vi "getAdditionalDataXML.vi"(8 "error in (no error)":errorcluster, 11 "PlayFile in":refnum<class "PlayFile.lvclass">) -> (0 "error out":errorcluster, 2 "additionalDataXML":refnum<class "xmlNode.lvclass">, 3 "PlayFile out":refnum<class "PlayFile.lvclass">)   [LabVIEW 2011, in "Tools.lvlib" / "Scripting.lvlib" / "PlayFile.lvclass"]
uses:
  PlayFile.lvclass
  xmlNode/xmlNode.lvclass
  PlayFile.lvclass/PlayFile.ctl
  ScriptEvent.lvclass
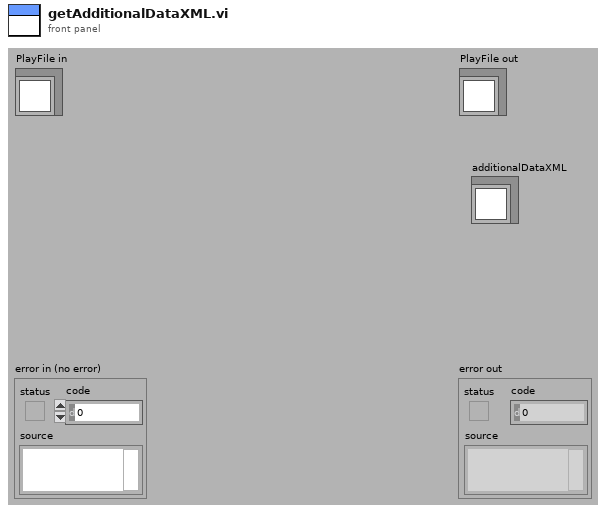
[diagram p1: front panel]
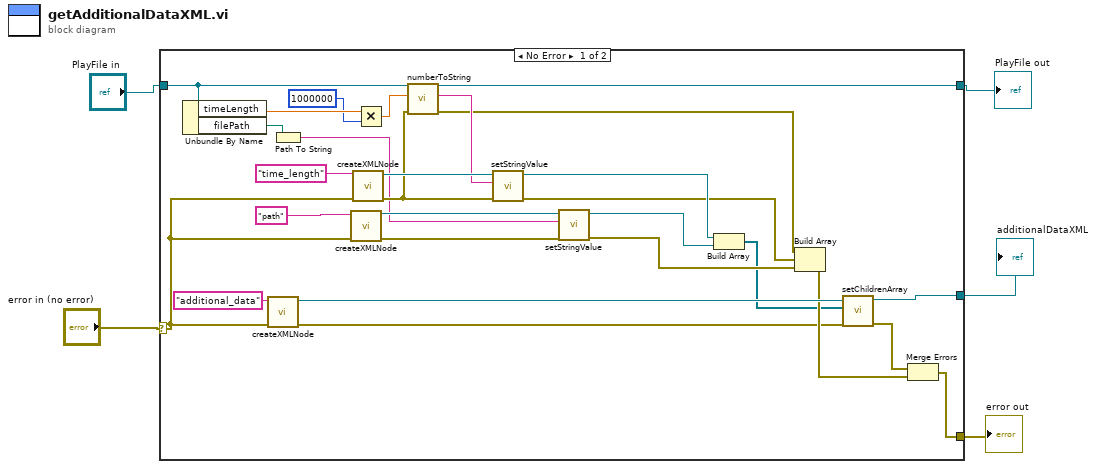
[diagram p0: block diagram]
diagram:
  n1 = case shown="No Error" "error in (no error)" {
    selector: "error in (no error)" -> [w31 w34]
    tunnel: "PlayFile in" -> [w14 w35]
    tunnel: [w7 w35] -> w1
    tunnel: [w18 w34] -> w2
    tunnel: [w17 _] -> w3
    frame No Error {
      n2 = Unbundle By Name(w14) -> ("timeLength"=w30:dbl, "filePath"=w10:path)
      n3 = call "createXMLNode.vi"("error in (no error)"=w31, "name"="additional_data") -> ("error out"=w15:errorcluster, "xmlNode out"=w21:refnum<class "xmlNode.lvclass">)  [unwired: 8 in]
      n4 = Path To String(path=w10) -> (string=w9:string)
      n5 = call "createXMLNode.vi"("error in (no error)"=w31, "name"="path") -> ("error out"=w26:errorcluster, "xmlNode out"=w27:refnum<class "xmlNode.lvclass">)  [unwired: 8 in]
      n6 = call "createXMLNode.vi"("error in (no error)"=w31, "name"="time_length") -> ("error out"=w11:errorcluster, "xmlNode out"=w28:refnum<class "xmlNode.lvclass">)  [unwired: 8 in]
      n7 = Multiply(x=w30, y=1000000) -> (x*y=w13:dbl)
      n8 = call "numberToString.vi"("error in (no error)"=w11, "Numeric"=w13, "ScriptEvent in"=w14) -> ("error out"=w6:errorcluster, "String"=w12:string, "ScriptEvent out"=w7:refnum<class "PlayFile.lvclass">)  [unwired: 6 in]
      n9 = call-dynamic "setStringValue.vi"("error in (no error)"=w11, "stringValue"=w12, "xmlNode.lvclass in"=w28) -> ("error out"=w23:errorcluster, "xmlNode.lvclass out"=w25:refnum<class "xmlNode.lvclass">)  [unwired: 7 in]
      n10 = call-dynamic "setStringValue.vi"("error in (no error)"=w26, "stringValue"=w9, "xmlNode.lvclass in"=w27) -> ("error out"=w22:errorcluster, "xmlNode.lvclass out"=w24:refnum<class "xmlNode.lvclass">)  [unwired: 7 in]
      n11 = Build Array(w25, w24) -> (w8:refnum<class "xmlNode.lvclass">[])
      n12 = Build Array(w6, w23, w22) -> (w19:errorcluster[])
      n13 = call-dynamic "setChildrenArray.vi"("error in (no error)"=w15, "Children"=w8, "xmlNode.lvclass in"=w21) -> ("error out"=w20:errorcluster, "xmlNode.lvclass out"=w17:refnum<class "xmlNode.lvclass">)  [unwired: 7 in]
      n14 = Merge Errors(w20, w19) -> (w18:errorcluster)
    }
    frame Error {
    }
  }
  "error out" <- w2
  "PlayFile out" <- w1
  "additionalDataXML" <- w3
